vi "Create.vi"(10 "display ref":refnum<vi>) -> (3 "Sudoku.lvclass out":refnum<class "Sudoku.lvclass">)   [LabVIEW 2021, in "Sudoku.lvclass"]
uses:
  Sudoku.lvclass
  Sudoku.lvclass/Sudoku.ctl
  Cell/Cell.lvclass
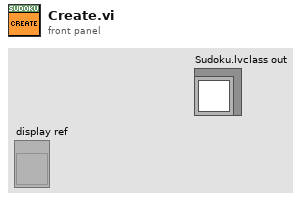
[diagram p1: front panel]
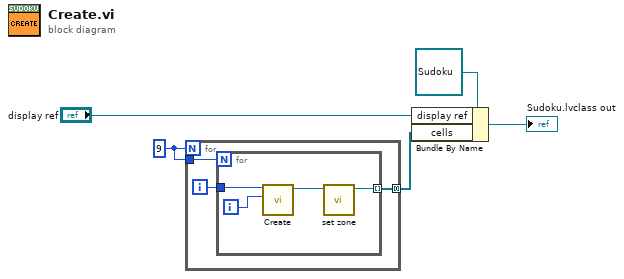
[diagram p0: block diagram]
diagram:
  w2 = 9
  n1 = for {
    N: w2 -> [_]
    tunnel: w2 -> [w8]
    tunnel: [w6] -> w1 mode=concatenating
    i -> [w7]
    n2 = for {
      N: w8 -> [_]
      tunnel: w7 -> [w12]
      tunnel: [w9] -> w6 mode=indexing
      i -> [w11]
      n3 = call "Create.vi"("col"=w11, "row"=w12) -> ("output cluster"=w10:refnum<class "Cell.lvclass">)  [unwired: 9 in]
      n4 = call "set zone.vi"("Cell.lvclass in"=w10) -> ("Cell.lvclass out"=w9:refnum<class "Cell.lvclass">)  [unwired: 10 in]
    }
  }
  n5 = Bundle By Name(cluster=refnum<class "Sudoku.lvclass"> refnum ("Sudoku.lvclass"), "display ref"="display ref", "cells"=w1) -> (→"Sudoku.lvclass out":refnum<class "Sudoku.lvclass">)
